vi "Get Daemon Connection Count.vi"(8 "error in (no error)":errorcluster, 11 "Modbus slave in":refnum<class "Modbus Slave.lvclass">) -> (0 "error out":errorcluster, 2 "connection count":u32, 3 "Modbus slave out":refnum<class "Modbus Slave.lvclass">)   [LabVIEW 2020, in "Modbus Slave.lvclass"]
doc: "<B>TCP Connection Count</B> returns the number of TCP connections established to the Modbus slave. This property indicates the number of Modbus masters connected to the Modbus slave. To get this property, ensure that you wire a TCP Modbus slave to the <B>reference</B> input. Otherwise, LabVIEW returns error code -389106."
uses:
  <vilib>/Modbus/slave/Modbus Slave.lvclass
  <vilib>/Modbus/slave/Modbus Slave.lvclass/Modbus Slave.ctl
  <vilib>/Modbus/subvis/Protocol/TCP/TCP Slave/TCP Slave.lvclass
  <vilib>/Modbus/subvis/Protocol/TCP/TCP Slave/TCP Slave.lvclass/TCP Slave.ctl
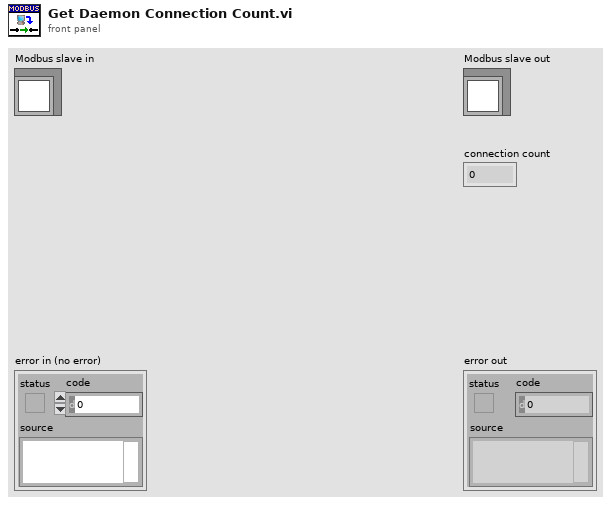
[diagram p1: front panel]
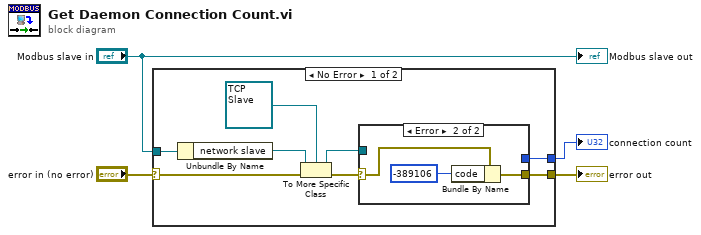
[diagram p0: block diagram]
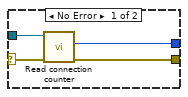
[diagram p2: hidden frame]
diagram:
  n1 = case shown="No Error" "error in (no error)" {
    selector: "error in (no error)" -> [w11 w20]
    tunnel: [w8 _] -> w3
    tunnel: [w7 w20] -> w2
    tunnel: "Modbus slave in" -> [w5 _]
    frame No Error {
      n2 = Unbundle By Name(w5) -> ("network slave"=w6:refnum<class "Network Slave.lvclass">)
      n3 = To More Specific Class(target class=refnum<class "TCP Slave.lvclass"> refnum ("TCP Slave"), reference=w6, error in=w11) -> (specific class reference=w9:refnum<class "TCP Slave.lvclass">, error out=w10:errorcluster)
      n4 = case shown="Error" w10 {
        selector: w10 -> [w15 w19]
        tunnel: w9 -> [w16 _]
        tunnel: [w13 _] -> w8
        tunnel: [w14 w18] -> w7
        frame No Error {
          n5 = call <vilib>:"Read connection counter.vi"("error in (no error)"=w15, "TCP slave in"=w16) -> ("error out"=w14:errorcluster, "currently connected"=w13:u32)  [unwired: 7 in, 1 out]
        }
        frame Error {
          n6 = Bundle By Name(cluster=w19, "code"=-389106) -> (w18:errorcluster)
        }
      }
    }
    frame Error {
    }
  }
  "error out" <- w2
  "connection count" <- w3
  "Modbus slave out" <- "Modbus slave in"
